vi "LWXPS_EventExtendedConfigurationTriggerGet.vi"(0 "XPS Reference IN":refnum<k24>, 11 "LabVIEW error IN":errorcluster) -> (4 "XPS Reference OUT":refnum<k24>, 6 "Returned error code":i32, 8 "Event Trigger Configuration":string, 10 "XPS Error String":string, 15 "LabVIEW error OUT":errorcluster)   [LabVIEW 2014]
uses:
  D:/XPSQ8_LabView_Library/Development/Source/Dll/Newport.XPS.CommandInterface.dll
  Dll/Newport.XPS.CommandInterface.dll
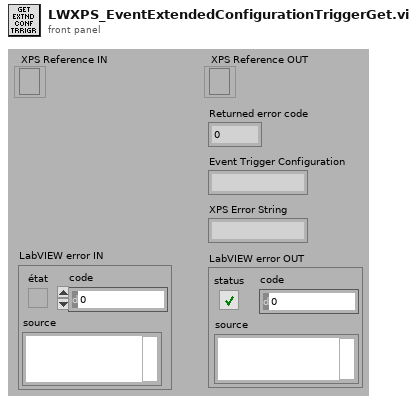
[diagram p1: front panel]
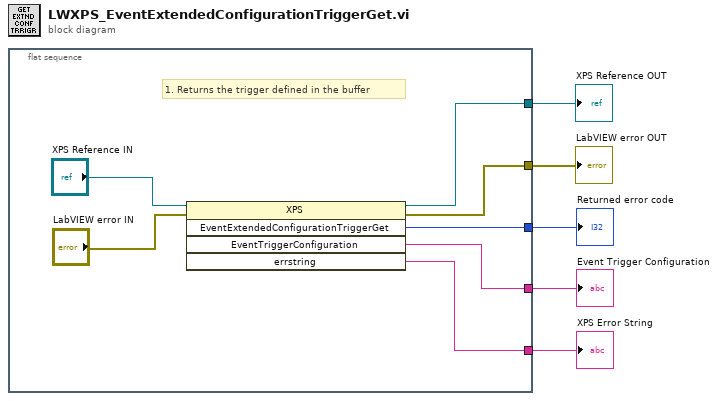
[diagram p0: block diagram]
diagram:
  n1 = flat-sequence {
    tunnel: [w6] -> w1
    tunnel: [w10] -> w3
    tunnel: [w9] -> w5
    tunnel: [w8] -> w4
    tunnel: [w7] -> w2
    frame #0 {
      # "1. Returns the trigger defined in the buffer"
      n2 = invoke class="XPS" method="EventExtendedConfigurationTriggerGet"(reference="XPS Reference IN", error in="LabVIEW error IN") -> (reference out=w9:refnum<k24>, error out=w8:errorcluster, "EventExtendedConfigurationTriggerGet"=w7:i32, "EventTriggerConfiguration"=w6:string, "errstring"=w10:string)  [unwired: 3 in]
    }
  }
  "XPS Reference OUT" <- w5
  "LabVIEW error OUT" <- w4
  "XPS Error String" <- w3
  "Returned error code" <- w2
  "Event Trigger Configuration" <- w1
